vi "Configuration Convert 1.3 to 1.4.vi"(8 "error in (no error)":errorcluster, 11 "configuration 1.3":T2) -> (0 "error out":errorcluster, 3 "configuration 1.4":T1)   [LabVIEW 2021, in "DSF Core.lvlib" / "Configuration Session.lvclass"]
uses:
  Configuration Session.lvclass
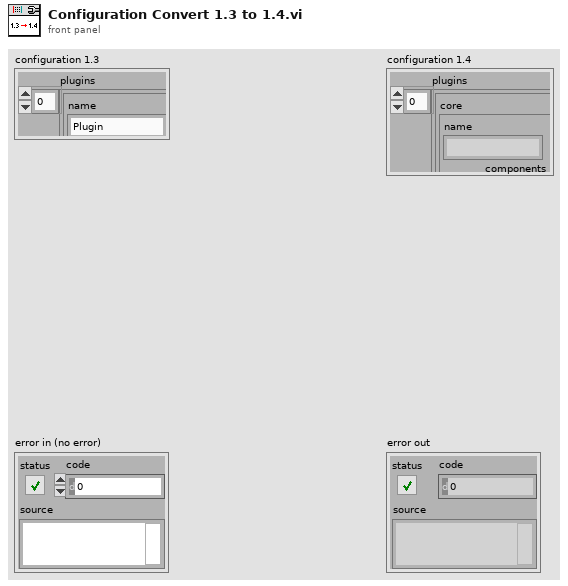
[diagram p1: front panel]
types:
  T1 = cluster{"plugins":cluster{"core":cluster{"name":string, "components":string[], "cycle timing":cluster{"priority":u64, "decimation":u64, "offset":u64}}, "component settings":cluster{"component":string, "values":cluster{"key":string, "value":string}[]}[], "threads":cluster{"core":cluster{"processor":i32, "priority offset":i16}, "component settings":cluster{"component":string, "values":cluster{"key":string, "value":string}[]}[], "transfer groups":cluster{"core":cluster{"name":string, "direction":enum8{"Tx", "Rx"}, "cycle timing":cluster{"priority":u64, "decimation":u64, "offset":u64}, "timeout behavior":enum8{"Increment Late Count", "Throw Error"}, "enable conversion":bool}, "component settings":cluster{"component":string, "values":cluster{"key":string, "value":string}[]}[], "transfers":cluster{"core":cluster{"name":string}, "component settings":cluster{"component":string, "values":cluster{"key":string, "value":string}[]}[], "channels":cluster{"core":cluster{"name":string, "units":string, "engine data type":enum8{"Bool", "SGL", "DBL", "I8", "I16", "I32", "I64", "U8", "U16", "U32", "U64"}, "string data type":enum8{"Bool", "SGL", "DBL", "I8", "I16", "I32", "I64", "U8", "U16", "U32", "U64"}, "string offset":u64}, "component settings":cluster{"component":string, "values":cluster{"key":string, "value":string}[]}[]}[]}[]}[]}[]}[]}
  T2 = cluster{"plugins":cluster{"name":string, "components":string[], "cycle timing":cluster{"priority":u64, "decimation":u64, "offset":u64}, "threads":cluster{"processor":i32, "priority offset":i16, "settings":cluster{"component":string, "name":string, "values":cluster{"key":string, "value":string}[]}[]}[], "transfer groups":cluster{"name":string, "direction":enum8{"Tx", "Rx"}, "cycle timing":cluster{"priority":u64, "decimation":u64, "offset":u64}, "thread index":u8, "settings":cluster{"component":string, "name":string, "values":cluster{"key":string, "value":string}[]}[], "transfers":cluster{"name":string, "byte order":enum8{"big-endian", "little-endian"}, "settings":cluster{"component":string, "name":string, "values":cluster{"key":string, "value":string}[]}[], "channels":cluster{"string offset":u64, "name":string, "units":string, "engine data type":enum8{"Bool", "SGL", "DBL", "I8", "I16", "I32", "I64", "U8", "U16", "U32", "U64"}, "string data type":enum8{"Bool", "SGL", "DBL", "I8", "I16", "I32", "I64", "U8", "U16", "U32", "U64"}, "settings":cluster{"component":string, "name":string, "values":cluster{"key":string, "value":string}[]}[]}[]}[], "timeout behavior":enum8{"Increment Late Count", "Throw Error"}, "enable buffer conversion":bool}[], "settings":cluster{"component":string, "name":string, "values":cluster{"key":string, "value":string}[]}[]}[]}
  T3 = cluster{"core":cluster{"name":string, "components":string[], "cycle timing":cluster{"priority":u64, "decimation":u64, "offset":u64}}, "component settings":cluster{"component":string, "values":cluster{"key":string, "value":string}[]}[], "threads":cluster{"core":cluster{"processor":i32, "priority offset":i16}, "component settings":cluster{"component":string, "values":cluster{"key":string, "value":string}[]}[], "transfer groups":cluster{"core":cluster{"name":string, "direction":enum8{"Tx", "Rx"}, "cycle timing":cluster{"priority":u64, "decimation":u64, "offset":u64}, "timeout behavior":enum8{"Increment Late Count", "Throw Error"}, "enable conversion":bool}, "component settings":cluster{"component":string, "values":cluster{"key":string, "value":string}[]}[], "transfers":cluster{"core":cluster{"name":string}, "component settings":cluster{"component":string, "values":cluster{"key":string, "value":string}[]}[], "channels":cluster{"core":cluster{"name":string, "units":string, "engine data type":enum8{"Bool", "SGL", "DBL", "I8", "I16", "I32", "I64", "U8", "U16", "U32", "U64"}, "string data type":enum8{"Bool", "SGL", "DBL", "I8", "I16", "I32", "I64", "U8", "U16", "U32", "U64"}, "string offset":u64}, "component settings":cluster{"component":string, "values":cluster{"key":string, "value":string}[]}[]}[]}[]}[]}[]}
  T4 = cluster{"core":cluster{"processor":i32, "priority offset":i16}, "component settings":cluster{"component":string, "values":cluster{"key":string, "value":string}[]}[], "transfer groups":cluster{"core":cluster{"name":string, "direction":enum8{"Tx", "Rx"}, "cycle timing":cluster{"priority":u64, "decimation":u64, "offset":u64}, "timeout behavior":enum8{"Increment Late Count", "Throw Error"}, "enable conversion":bool}, "component settings":cluster{"component":string, "values":cluster{"key":string, "value":string}[]}[], "transfers":cluster{"core":cluster{"name":string}, "component settings":cluster{"component":string, "values":cluster{"key":string, "value":string}[]}[], "channels":cluster{"core":cluster{"name":string, "units":string, "engine data type":enum8{"Bool", "SGL", "DBL", "I8", "I16", "I32", "I64", "U8", "U16", "U32", "U64"}, "string data type":enum8{"Bool", "SGL", "DBL", "I8", "I16", "I32", "I64", "U8", "U16", "U32", "U64"}, "string offset":u64}, "component settings":cluster{"component":string, "values":cluster{"key":string, "value":string}[]}[]}[]}[]}[]}
  T5 = cluster{"component":string, "values":cluster{"key":string, "value":string}[]}
  T6 = cluster{"core":cluster{"name":string, "direction":enum8{"Tx", "Rx"}, "cycle timing":cluster{"priority":u64, "decimation":u64, "offset":u64}, "timeout behavior":enum8{"Increment Late Count", "Throw Error"}, "enable conversion":bool}, "component settings":cluster{"component":string, "values":cluster{"key":string, "value":string}[]}[], "transfers":cluster{"core":cluster{"name":string}, "component settings":cluster{"component":string, "values":cluster{"key":string, "value":string}[]}[], "channels":cluster{"core":cluster{"name":string, "units":string, "engine data type":enum8{"Bool", "SGL", "DBL", "I8", "I16", "I32", "I64", "U8", "U16", "U32", "U64"}, "string data type":enum8{"Bool", "SGL", "DBL", "I8", "I16", "I32", "I64", "U8", "U16", "U32", "U64"}, "string offset":u64}, "component settings":cluster{"component":string, "values":cluster{"key":string, "value":string}[]}[]}[]}[]}
  T7 = cluster{"core":cluster{"name":string}, "component settings":cluster{"component":string, "values":cluster{"key":string, "value":string}[]}[], "channels":cluster{"core":cluster{"name":string, "units":string, "engine data type":enum8{"Bool", "SGL", "DBL", "I8", "I16", "I32", "I64", "U8", "U16", "U32", "U64"}, "string data type":enum8{"Bool", "SGL", "DBL", "I8", "I16", "I32", "I64", "U8", "U16", "U32", "U64"}, "string offset":u64}, "component settings":cluster{"component":string, "values":cluster{"key":string, "value":string}[]}[]}[]}
  T8 = cluster{"core":cluster{"name":string, "units":string, "engine data type":enum8{"Bool", "SGL", "DBL", "I8", "I16", "I32", "I64", "U8", "U16", "U32", "U64"}, "string data type":enum8{"Bool", "SGL", "DBL", "I8", "I16", "I32", "I64", "U8", "U16", "U32", "U64"}, "string offset":u64}, "component settings":cluster{"component":string, "values":cluster{"key":string, "value":string}[]}[]}
  T9 = cluster{"name":string, "components":string[], "cycle timing":cluster{"priority":u64, "decimation":u64, "offset":u64}, "threads":cluster{"processor":i32, "priority offset":i16, "settings":cluster{"component":string, "name":string, "values":cluster{"key":string, "value":string}[]}[]}[], "transfer groups":cluster{"name":string, "direction":enum8{"Tx", "Rx"}, "cycle timing":cluster{"priority":u64, "decimation":u64, "offset":u64}, "thread index":u8, "settings":cluster{"component":string, "name":string, "values":cluster{"key":string, "value":string}[]}[], "transfers":cluster{"name":string, "byte order":enum8{"big-endian", "little-endian"}, "settings":cluster{"component":string, "name":string, "values":cluster{"key":string, "value":string}[]}[], "channels":cluster{"string offset":u64, "name":string, "units":string, "engine data type":enum8{"Bool", "SGL", "DBL", "I8", "I16", "I32", "I64", "U8", "U16", "U32", "U64"}, "string data type":enum8{"Bool", "SGL", "DBL", "I8", "I16", "I32", "I64", "U8", "U16", "U32", "U64"}, "settings":cluster{"component":string, "name":string, "values":cluster{"key":string, "value":string}[]}[]}[]}[], "timeout behavior":enum8{"Increment Late Count", "Throw Error"}, "enable buffer conversion":bool}[], "settings":cluster{"component":string, "name":string, "values":cluster{"key":string, "value":string}[]}[]}[]
  T10 = cluster{"priority":u64, "decimation":u64, "offset":u64}
  T11 = cluster{"component":string, "name":string, "values":cluster{"key":string, "value":string}[]}[]
  T12 = cluster{"processor":i32, "priority offset":i16, "settings":cluster{"component":string, "name":string, "values":cluster{"key":string, "value":string}[]}[]}[]
  T13 = cluster{"name":string, "direction":enum8{"Tx", "Rx"}, "cycle timing":cluster{"priority":u64, "decimation":u64, "offset":u64}, "thread index":u8, "settings":cluster{"component":string, "name":string, "values":cluster{"key":string, "value":string}[]}[], "transfers":cluster{"name":string, "byte order":enum8{"big-endian", "little-endian"}, "settings":cluster{"component":string, "name":string, "values":cluster{"key":string, "value":string}[]}[], "channels":cluster{"string offset":u64, "name":string, "units":string, "engine data type":enum8{"Bool", "SGL", "DBL", "I8", "I16", "I32", "I64", "U8", "U16", "U32", "U64"}, "string data type":enum8{"Bool", "SGL", "DBL", "I8", "I16", "I32", "I64", "U8", "U16", "U32", "U64"}, "settings":cluster{"component":string, "name":string, "values":cluster{"key":string, "value":string}[]}[]}[]}[], "timeout behavior":enum8{"Increment Late Count", "Throw Error"}, "enable buffer conversion":bool}[]
  T14 = cluster{"name":string, "byte order":enum8{"big-endian", "little-endian"}, "settings":cluster{"component":string, "name":string, "values":cluster{"key":string, "value":string}[]}[], "channels":cluster{"string offset":u64, "name":string, "units":string, "engine data type":enum8{"Bool", "SGL", "DBL", "I8", "I16", "I32", "I64", "U8", "U16", "U32", "U64"}, "string data type":enum8{"Bool", "SGL", "DBL", "I8", "I16", "I32", "I64", "U8", "U16", "U32", "U64"}, "settings":cluster{"component":string, "name":string, "values":cluster{"key":string, "value":string}[]}[]}[]}[]
  T15 = cluster{"string offset":u64, "name":string, "units":string, "engine data type":enum8{"Bool", "SGL", "DBL", "I8", "I16", "I32", "I64", "U8", "U16", "U32", "U64"}, "string data type":enum8{"Bool", "SGL", "DBL", "I8", "I16", "I32", "I64", "U8", "U16", "U32", "U64"}, "settings":cluster{"component":string, "name":string, "values":cluster{"key":string, "value":string}[]}[]}[]
  T16 = enum8{"Bool", "SGL", "DBL", "I8", "I16", "I32", "I64", "U8", "U16", "U32", "U64"}
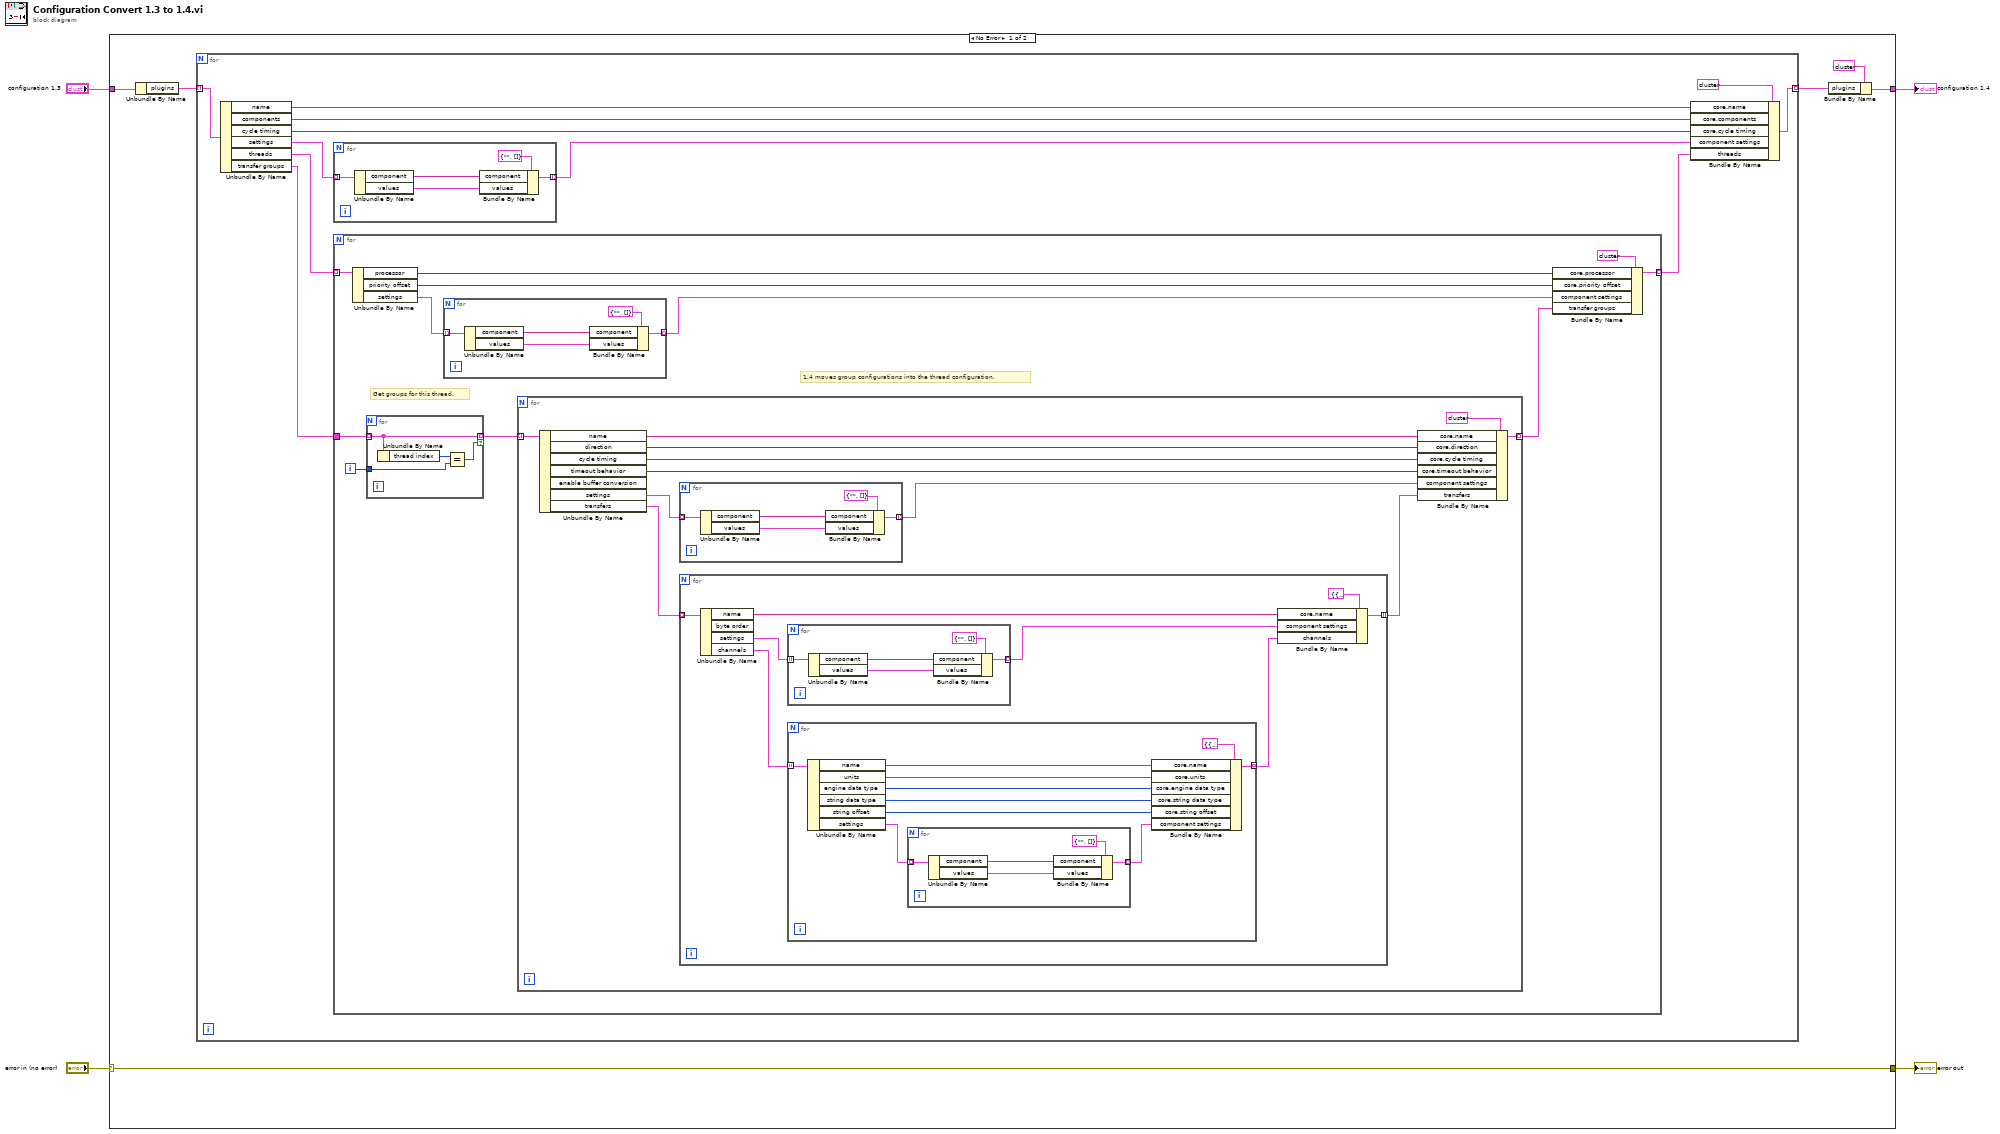
[diagram p0: block diagram]
diagram:
  n1 = case shown="No Error" "error in (no error)" {
    selector: "error in (no error)" -> [w10 w91]
    tunnel: [w10 w91] -> w4
    tunnel: "configuration 1.3" -> [w9 _]
    tunnel: [w8 _] -> w1
    frame No Error {
      n2 = Unbundle By Name(w9) -> ("plugins"=w7:T9)
      n3 = for {
        tunnel: w7 -> [w20] mode=indexing
        tunnel: [w17] -> w6 mode=indexing
        n4 = Unbundle By Name(w20) -> ("name"=w21:string, "components"=w19:string[], "cycle timing"=w18:T10, "settings"=w15:T11, "threads"=w14:T12, "transfer groups"=w13:T13)
        n5 = for {
          tunnel: w15 -> [w90] mode=indexing
          tunnel: [w87] -> w16 mode=indexing
          n6 = Unbundle By Name(w90) -> ("component"=w88:string, "values"=w86:cluster{"key":string, "value":string}[])
          n7 = Bundle By Name(cluster=T5 {"component"="", "values"=[]} ("settings 2"), "component"=w88, "values"=w86) -> (w87:T5)
        }
        n8 = for {
          tunnel: w14 -> [w32] mode=indexing
          tunnel: w13 -> [w26]
          tunnel: [w30] -> w12 mode=indexing
          i -> [w25]
          # "1.4 moves group configurations into the thread configuration."
          # "Get groups for this thread."
          n9 = Unbundle By Name(w32) -> ("processor"=w29:i32, "priority offset"=w28:i16, "settings"=w31:T11)
          n10 = for {
            tunnel: w26 -> [w84] mode=indexing
            tunnel: w25 -> [w85]
            tunnel: [w84] -> w24 mode=indexing if=w83
            n11 = Unbundle By Name(w84) -> ("thread index"=w82:u8)
            n12 = Equal?(x=w82, y=w85) -> (x = y?=w83:bool)
          }
          n13 = for {
            tunnel: w31 -> [w37] mode=indexing
            tunnel: [w34] -> w27 mode=indexing
            n14 = Unbundle By Name(w37) -> ("component"=w35:string, "values"=w33:cluster{"key":string, "value":string}[])
            n15 = Bundle By Name(cluster=T5 {"component"="", "values"=[]} ("settings 2"), "component"=w35, "values"=w33) -> (w34:T5)
          }
          n16 = for {
            tunnel: w24 -> [w48] mode=indexing
            tunnel: [w47] -> w23 mode=indexing
            n17 = Unbundle By Name(w48) -> ("name"=w46:string, "direction"=w45:enum8{"Tx", "Rx"}, "cycle timing"=w44:T10, "timeout behavior"=w43:enum8{"Increment Late Count", "Throw Error"}, "settings"=w42:T11, "transfers"=w40:T14)  [unwired: 1 out]
            n18 = for {
              tunnel: w42 -> [w81] mode=indexing
              tunnel: [w78] -> w41 mode=indexing
              n19 = Unbundle By Name(w81) -> ("component"=w79:string, "values"=w77:cluster{"key":string, "value":string}[])
              n20 = Bundle By Name(cluster=T5 {"component"="", "values"=[]} ("settings 2"), "component"=w79, "values"=w77) -> (w78:T5)
            }
            n21 = for {
              tunnel: w40 -> [w55] mode=indexing
              tunnel: [w56] -> w39 mode=indexing
              n22 = Unbundle By Name(w55) -> ("name"=w54:string, "settings"=w53:T11, "channels"=w51:T15)  [unwired: 1 out]
              n23 = for {
                tunnel: w53 -> [w76] mode=indexing
                tunnel: [w74] -> w52 mode=indexing
                n24 = Unbundle By Name(w76) -> ("component"=w75:string, "values"=w73:cluster{"key":string, "value":string}[])
                n25 = Bundle By Name(cluster=T5 {"component"="", "values"=[]} ("settings 2"), "component"=w75, "values"=w73) -> (w74:T5)
              }
              n26 = for {
                tunnel: w51 -> [w66] mode=indexing
                tunnel: [w65] -> w50 mode=indexing
                n27 = Unbundle By Name(w66) -> ("name"=w64:string, "units"=w63:string, "engine data type"=w62:T16, "string data type"=w61:T16, "string offset"=w60:u64, "settings"=w59:T11)
                n28 = for {
                  tunnel: w59 -> [w71] mode=indexing
                  tunnel: [w68] -> w58 mode=indexing
                  n29 = Unbundle By Name(w71) -> ("component"=w69:string, "values"=w67:cluster{"key":string, "value":string}[])
                  n30 = Bundle By Name(cluster=T5 {"component"="", "values"=[]} ("settings 2"), "component"=w69, "values"=w67) -> (w68:T5)
                }
                n31 = Bundle By Name(cluster=T8 {"core"={"name"="Channel", "units"="V", "engine data type"=enum."DBL", "string data type"=enum."DBL", "string offset"=0}, "component settings"=[]} ("channel configuration"), "core.name"=w64, "core.units"=w63, "core.engine data type"=w62, "core.string data type"=w61, "core.string offset"=w60, "component settings"=w58) -> (w65:T8)
              }
              n32 = Bundle By Name(cluster=T7 {"core"={"name"="Transfer"}, "component settings"=[], "channels"=[{"core"={"name"="Channel", "units"="V", "engine data type"=enum."DBL", "string data type"=enum."DBL", "string offset"=0}, "component settings"=[]}]} ("transfers"), "core.name"=w54, "component settings"=w52, "channels"=w50) -> (w56:T7)
            }
            n33 = Bundle By Name(cluster=T6 {"core"={"name"="Group", "direction"=enum."Tx", "cycle timing"={"priority"=100, "decimation"=1, "offset"=0}, "timeout behavior"=enum."Increment Late Count", "enable conversion"=FALSE}, "component settings"=[], "transfers"=[{"core"={"name"="Transfer"}, "component settings"=[], "channels"=[{"core"={"name"="Channel", "units"="V", "engine data type"=enum."DBL", "string data type"=enum."DBL", "string offset"=0}, "component settings"=[]}]}]} ("Transfer Group Configuration"), "core.name"=w46, "core.direction"=w45, "core.cycle timing"=w44, "core.timeout behavior"=w43, "component settings"=w41, "transfers"=w39) -> (w47:T6)
          }
          n34 = Bundle By Name(cluster=T4 {"core"={"processor"=-2, "priority offset"=0}, "component settings"=[], "transfer groups"=[{"core"={"name"="Group", "direction"=enum."Tx", "cycle timing"={"priority"=100, "decimation"=1, "offset"=0}, "timeout behavior"=enum."Increment Late Count", "enable conversion"=FALSE}, "component settings"=[], "transfers"=[{"core"={"name"="Transfer"}, "component settings"=[], "channels"=[{"core"={"name"="Channel", "units"="V", "engine data type"=enum."DBL", "string data type"=enum."DBL", "string offset"=0}, "component settings"=[]}]}]}]} ("threads"), "core.processor"=w29, "core.priority offset"=w28, "component settings"=w27, "transfer groups"=w23) -> (w30:T4)
        }
        n35 = Bundle By Name(cluster=T3 {"core"={"name"="", "components"=[], "cycle timing"={"priority"=10000, "decimation"=1, "offset"=0}}, "component settings"=[], "threads"=[{"core"={"processor"=-2, "priority offset"=0}, "component settings"=[], "transfer groups"=[{"core"={"name"="Group", "direction"=enum."Tx", "cycle timing"={"priority"=100, "decimation"=1, "offset"=0}, "timeout behavior"=enum."Increment Late Count", "enable conversion"=FALSE}, "component settings"=[], "transfers"=[{"core"={"name"="Transfer"}, "component settings"=[], "channels"=[{"core"={"name"="Channel", "units"="V", "engine data type"=enum."DBL", "string data type"=enum."DBL", "string offset"=0}, "component settings"=[]}]}]}]}]} ("Plugin Configuration"), "core.name"=w21, "core.components"=w19, "core.cycle timing"=w18, "component settings"=w16, "threads"=w12) -> (w17:T3)
      }
      n36 = Bundle By Name(cluster=T1 {"plugins"=[{"core"={"name"="", "components"=[], "cycle timing"={"priority"=10000, "decimation"=1, "offset"=0}}, "component settings"=[], "threads"=[{"core"={"processor"=-2, "priority offset"=0}, "component settings"=[], "transfer groups"=[{"core"={"name"="Group", "direction"=enum."Tx", "cycle timing"={"priority"=100, "decimation"=1, "offset"=0}, "timeout behavior"=enum."Increment Late Count", "enable conversion"=FALSE}, "component settings"=[], "transfers"=[{"core"={"name"="Transfer"}, "component settings"=[], "channels"=[{"core"={"name"="Channel", "units"="V", "engine data type"=enum."DBL", "string data type"=enum."DBL", "string offset"=0}, "component settings"=[]}]}]}]}]}]} ("configuration 1.4"), "plugins"=w6) -> (w8:T1)
    }
    frame Error {
    }
  }
  "error out" <- w4
  "configuration 1.4" <- w1
